vi "uActor_Core.vi"(8 "error in (no error)":errorcluster, 11 "uView in":refnum<class "uView.lvclass">) -> (0 "error out":errorcluster, 3 "uView out":refnum<class "uView.lvclass">)   [LabVIEW 2023, in "uFramework_pack_uActor.lvlib" / "uView.lvclass"]
uses:
  uView.lvclass
  uView.lvclass/uView.ctl
  uObserver/uObserver.lvclass
types:
  T1 = enum32{"Invalid", "Standard", "Closed", "Hidden", "Minimized", "Maximized"}
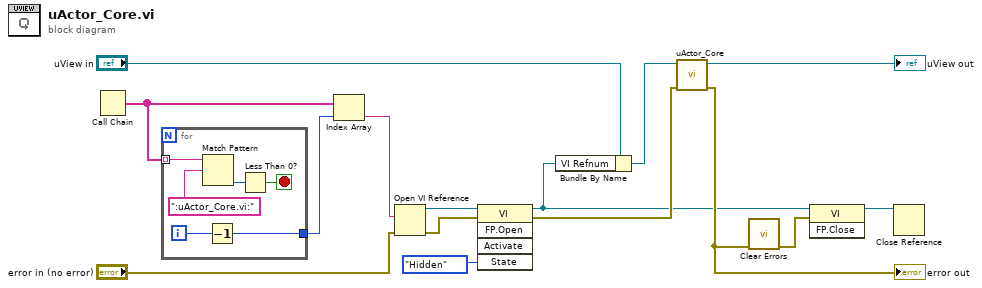
[diagram p0: block diagram]
diagram:
  n1 = Call Chain() -> (call chain=w13:string[])
  n2 = for {
    tunnel: w13 -> [w21] mode=indexing
    tunnel: [w17] -> w12
    i -> [w18]
    stop <- w16 stop-if-true
    n3 = Match Pattern(string=w21, regular expression=":uActor_Core.vi:") -> (offset past match=w19:i32)  [unwired: 1 in, 3 out]
    n4 = Decrement(x=w18) -> (x-1=w17:i32)
    n5 = Less Than 0?(x=w19) -> (x < 0?=w16:bool)
  }
  n6 = Index Array(array=w13, index=w12) -> (element=w11:string)
  n7 = Open VI Reference(vi path=w11, error in (no error)="error in (no error)") -> (vi reference=w10:refnum<vi>, error out=w4:errorcluster)  [unwired: 4 in]
  n8 = invoke class="VI" method="FP.Open"(reference=w10, error in=w4, "State"=T1."Hidden") -> (reference out=w1:refnum<vi>, error out=w15:errorcluster)  [unwired: 2 in, 3 out]
  n9 = Bundle By Name(cluster="uView in", "VI Refnum"=w1) -> (w8:refnum<class "uView.lvclass">)
  n10 = call-parent "uActor_Core.vi"("error in (no error)"=w15, "uActor in"=w8) -> ("error out"=w5:errorcluster, "uActor out"=→"uView out":refnum<class "uView.lvclass">)  [unwired: 8 in]
  "error out" <- w5
  n11 = call <vilib>:"Clear Errors.vi"("error in (no error)"=w5) -> ("error out"=w6:errorcluster)  [unwired: 5 in, 1 out]
  n12 = invoke class="VI" method="FP.Close"(reference=w1, error in=w6) -> (reference out=w2:refnum<vi>)  [unwired: 1 in, 2 out]
  n13 = Close Reference(reference=w2) -> ()  [unwired: 1 in, 1 out]
